vi "Close.vi"(8 "error in (no error)":errorcluster, 11 "MC switch refnum in":refnum<k24>) -> (0 "error out":errorcluster)   [LabVIEW 2019, in "Minicircuit RF Switch Box.lvlib"]
doc: "Terminaes the software connection to the instrument."
uses:
  <instrlib>/LV_Minicircuit_RF_Switch/Minicircuit RF Switch Box.lvlib
  C:/Program Files (x86)/National Instruments/LabVIEW 2019/instr.lib/LV_Minicircuit_RF_Switch/mcl_RF_Switch_Controller_NET45.dll
  mcl_RF_Switch_Controller_NET45.dll
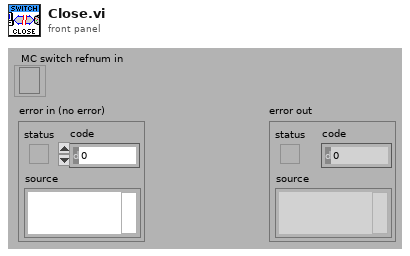
[diagram p1: front panel]
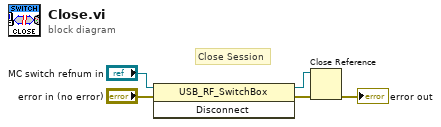
[diagram p0: block diagram]
diagram:
  # "Close Session"
  n1 = invoke class="USB_RF_SwitchBox" method="Disconnect"(reference="MC switch refnum in", error in="error in (no error)") -> (reference out=w2:refnum<k24>, error out=w1:errorcluster)  [unwired: 1 in, 1 out]
  n2 = Close Reference(reference=w2, error in (no error)=w1) -> (error out=→"error out":errorcluster)
